vi "CurrentFlow.vi"() -> ()   [LabVIEW 2012]
panel:
  in  "CurrentFlow":dbl
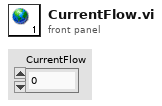
[diagram p1: front panel]
diagram:
